vi "总氮通讯.vi"() -> ()   [LabVIEW 2016, in "斯坦道总氮.lvlib"]
uses:
  <vilib>/NI/Modbus Library/API/Wrapper/Create TCP Slave.vi
  <vilib>/Utility/config.llb/Write Key (Boolean).vi
  <vilib>/Utility/config.llb/Write Key (String).vi
  <vilib>/Plasmionique/MB Master/MB_Master/MB_Master.lvclass
  <vilib>/NI/Modbus Library/API/Slave/Modbus Slave.lvclass
  <vilib>/Utility/config.llb/NI_LVConfig.lvlib
  <vilib>/Plasmionique/MB Master/MB Master.lvlib
  <vilib>/NI/Modbus Library/API/Wrapper/API Main.lvlib
panel:
  out "总氮测量数据区":u16[](array[numeric])
  out "总氮状态告警区":u16[](array[numeric])
  out "总磷状态告警区":u16[](array[numeric])
  out "总磷测量数据区":u16[](array[numeric])
  out "序列号":string
  out "状态告警区":T1 {"告警代码" items=["无告警", "缺试剂告警", "缺水样告警", "缺蒸馏水告警", "缺标液告警", "仪表漏液告警", "标定异常告警", "超量程告警", "加热异常", "低试剂预警", "超上限告警", "超下限告警", "仪表内部其他异常", "滴定异常告警", "电极异常告警", "量程切换告警", "参数设置告警", "PH电极电位异常", "电导率电极异常", "浊度光度异常", "溶解氧电极异常", "溶解氧光强异常", "温度异常告警", "PH异常告警", "溶解氧异常告警", "电导率异常告警", "浊度异常告警", "叶绿素异常告警", "藻密度异常告警", "蓝绿藻异常告警", "ORP异常告警", "氨氮异常告警", "清洁刷异常告警", "SD卡异常告警", "蓝牙异常告警", "Wifi异常告警", "流程异常告警"]; "故障代码" items=["无故障", "电机故障", "温度故障", "通讯故障", "滴定故障"]}
  out "测量数据区":T2 {"单位" items=["ug/L", "mg/L", "ppm", "mg/m3", "cm", "ppb", "ug/m3", "%", "nmol/mol", "umol/mol", "MPN/L", "MPN/100ml", "ng/m3", "NTU", "无量纲", "ms/cm", "us/cm", "℃", "mV", "万个/L"]}
  out "status":bool
  out "关键参数区":T3
  in  "读关键参数区":bool
  in  "读状态告警区":bool
  in  "读测量数据区":bool
  in  "站号":u16(ring) items=["总磷"=1, "氨氮"=3]
  in  "停止":bool
  in  "启动":bool
  in  "控制命令":u16(ring) items=["启动测量"=1, "标样核查"=2, "零点核查"=3, "跨度核查"=4, "空白测试"=5, "平行样测试"=6, "加标回收"=7, "空白校准"=8, "标样校准"=9, "初始化（清洗）"=10, "停止测试"=11, "仪器重启"=12, "校时"=13, "模式设置"=14, "测量间隔设置"=15]
  in  "控制命令参数":u16[](array[numeric]) format="%04xH"
  in  "VISA Resource":refnum<visa-resource-name>
  in  "启用模块":bool
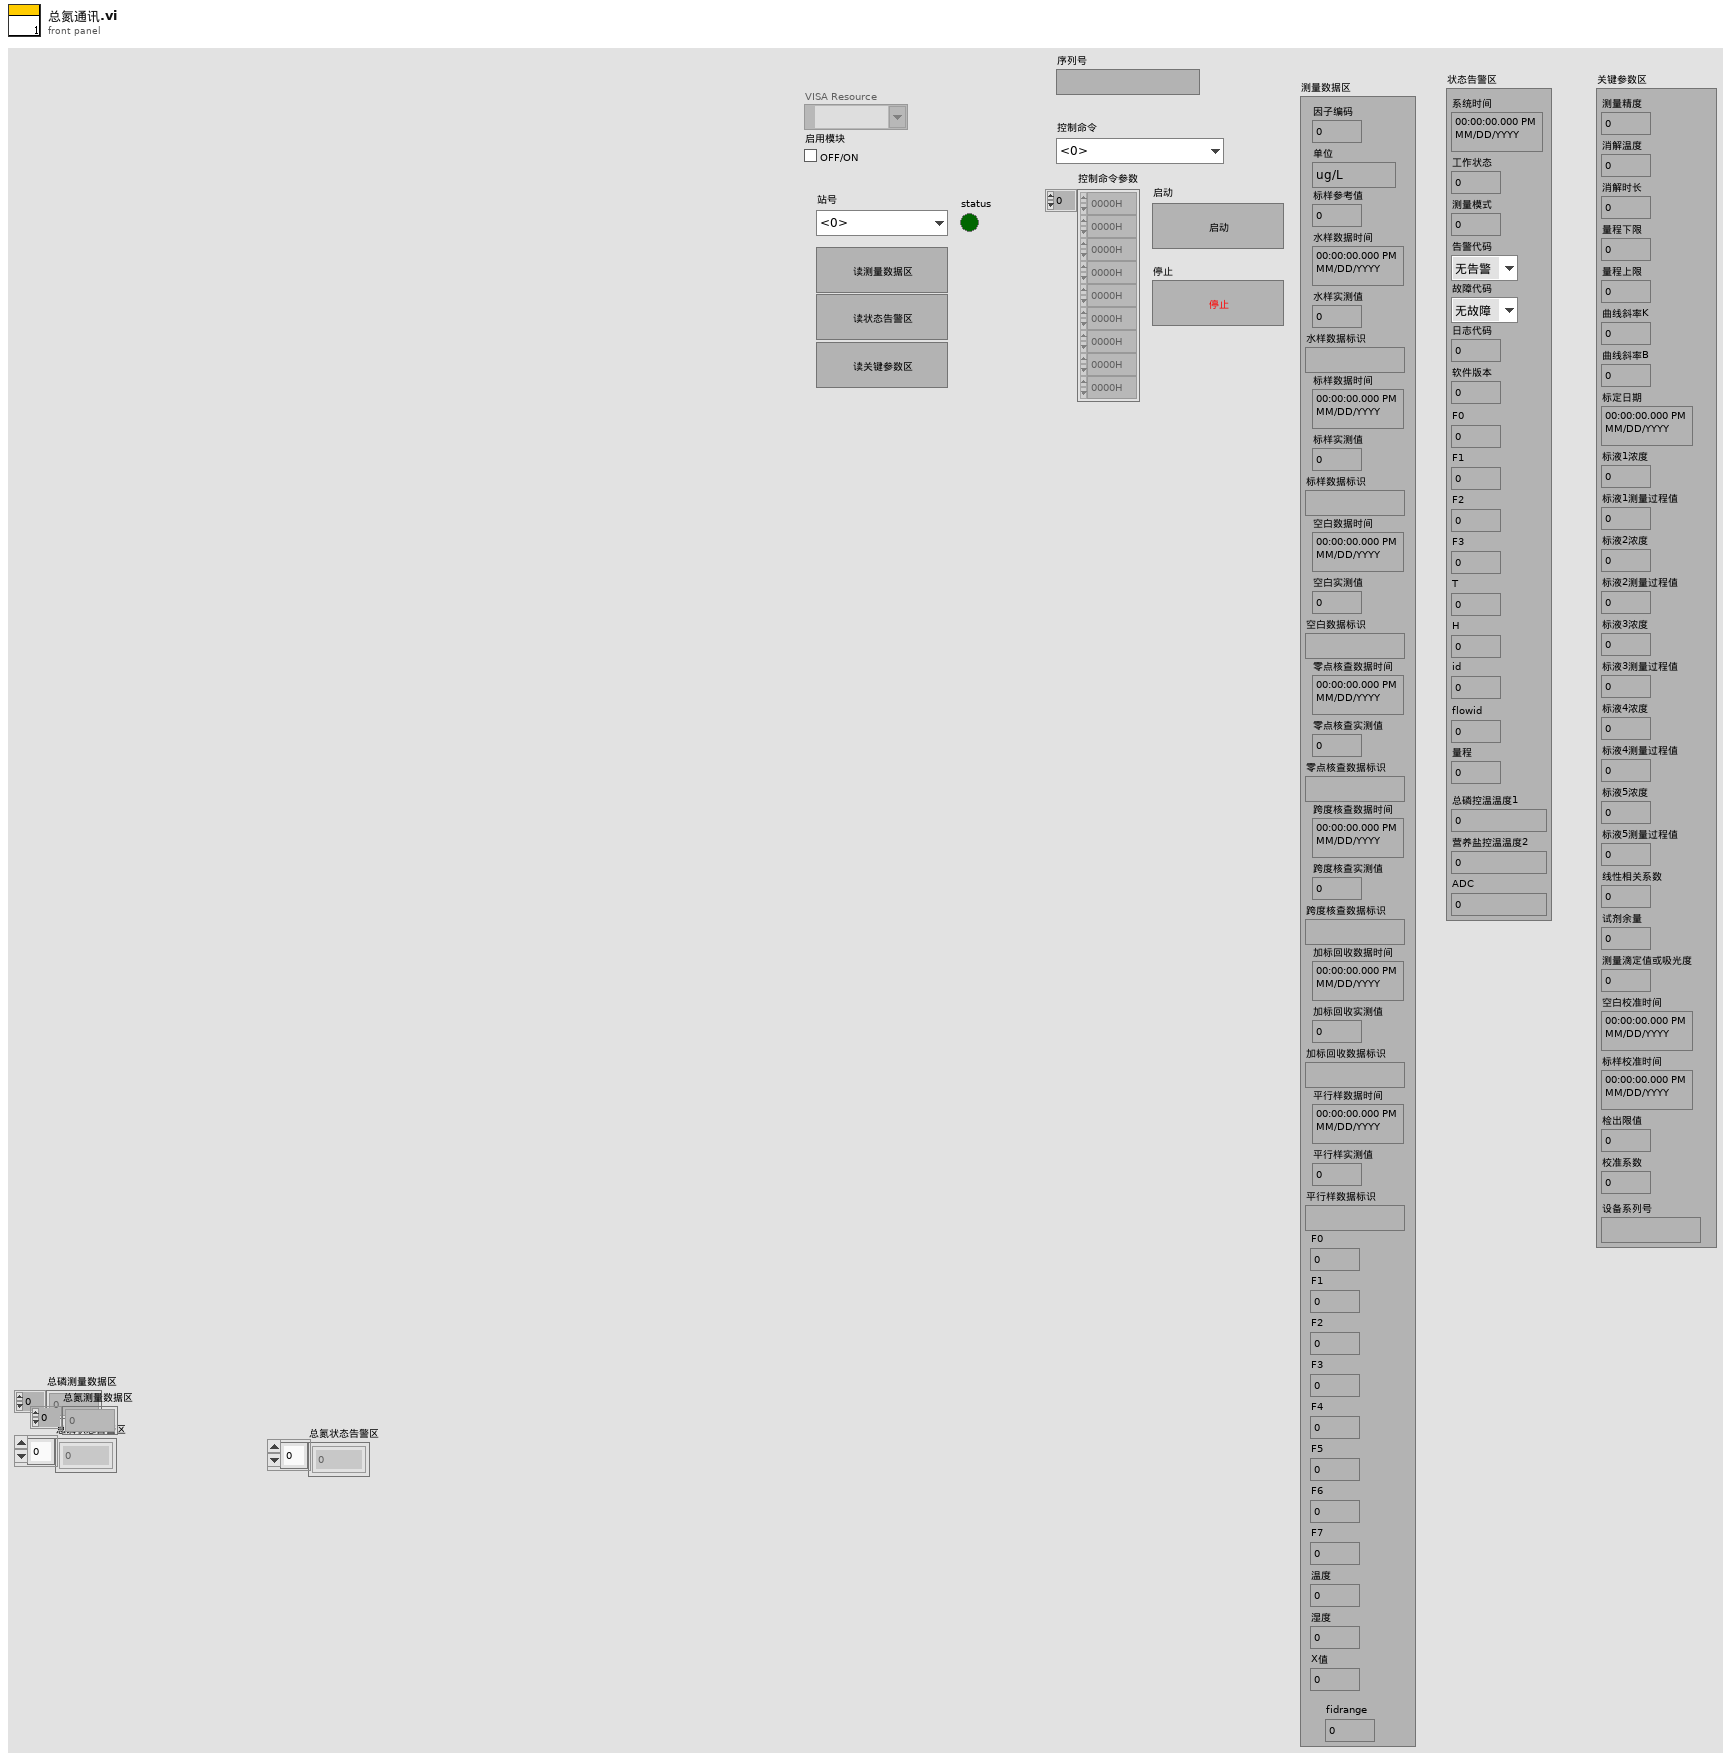
[diagram p1: front panel]
types:
  T1 = cluster{"系统时间":timestamp, "工作状态":u16, "测量模式":u16, "告警代码":u16, "故障代码":u16, "日志代码":u16, "软件版本":u16, "F0":sgl, "F1":sgl, "F2":sgl, "F3":sgl, "T":sgl, "H":sgl, "id":u16, "flowid":u16, "量程":u16, "总磷控温温度1":sgl, "营养盐控温温度2":sgl, "ADC":sgl}
  T2 = cluster{"因子编码":u32, "单位":u16, "标样参考值":sgl, "水样数据时间":timestamp, "水样实测值":sgl, "水样数据标识":string, "标样数据时间":timestamp, "标样实测值":sgl, "标样数据标识":string, "空白数据时间":timestamp, "空白实测值":sgl, "空白数据标识":string, "零点核查数据时间":timestamp, "零点核查实测值":sgl, "零点核查数据标识":string, "跨度核查数据时间":timestamp, "跨度核查实测值":sgl, "跨度核查数据标识":string, "加标回收数据时间":timestamp, "加标回收实测值":sgl, "加标回收数据标识":string, "平行样数据时间":timestamp, "平行样实测值":sgl, "平行样数据标识":string, "F0":sgl, "F1":sgl, "F2":sgl, "F3":sgl, "F4":sgl, "F5":sgl, "F6":sgl, "F7":sgl, "温度":sgl, "湿度":sgl, "X值":sgl, "fidrange":u16}
  T3 = cluster{"测量精度":u16, "消解温度":u16, "消解时长":u16, "量程下限":sgl, "量程上限":sgl, "曲线斜率K":sgl, "曲线斜率B":sgl, "标定日期":timestamp, "标液1浓度":sgl, "标液1测量过程值":sgl, "标液2浓度":sgl, "标液2测量过程值":sgl, "标液3浓度":sgl, "标液3测量过程值":sgl, "标液4浓度":sgl, "标液4测量过程值":sgl, "标液5浓度":sgl, "标液5测量过程值":sgl, "线性相关系数":sgl, "试剂余量":u32, "测量滴定值或吸光度":sgl, "空白校准时间":timestamp, "标样校准时间":timestamp, "检出限值":sgl, "校准系数":sgl, "设备系列号":string}
  T4 = cluster{"水样测试量程模式":enum16{"H", "L", "AUTO"}, "空白核查量程模式":enum16{"H", "L", "AUTO"}, "跨度核查量程模式":enum16{"H", "L", "AUTO"}, "加标回收量程模式":enum16{"H", "L", "AUTO"}}
  T5 = typedef "NI_LVConfig.lvlib/Config Data RefNum.ctl" = refnum<k1>
  T6 = enum8{"Enabled", "Disabled", "Disabled and Grayed Out"}
  T7 = cluster{"系统时间":timestamp, "工作状态":enum16{"空闲", "水样测试", "标样核查", "零点核查", "跨度核查", "空白测试", "平行样测试", "加标回收", "空白校准", "标样校准", "初始化（清洗）"}, "测量模式":enum16{"待机", "连续模式", "周期模式", "定点模式", "受控模式", "手动模式"}, "告警代码":u16, "故障代码":u16, "日志代码":u16, "软件版本":u16, "F0":sgl, "F1":sgl, "F2":sgl, "F3":sgl, "T":sgl, "H":sgl, "id":u16, "flowid":u16, "量程":u16, "总磷控温温度1":sgl, "营养盐控温温度2":sgl, "ADC":sgl}
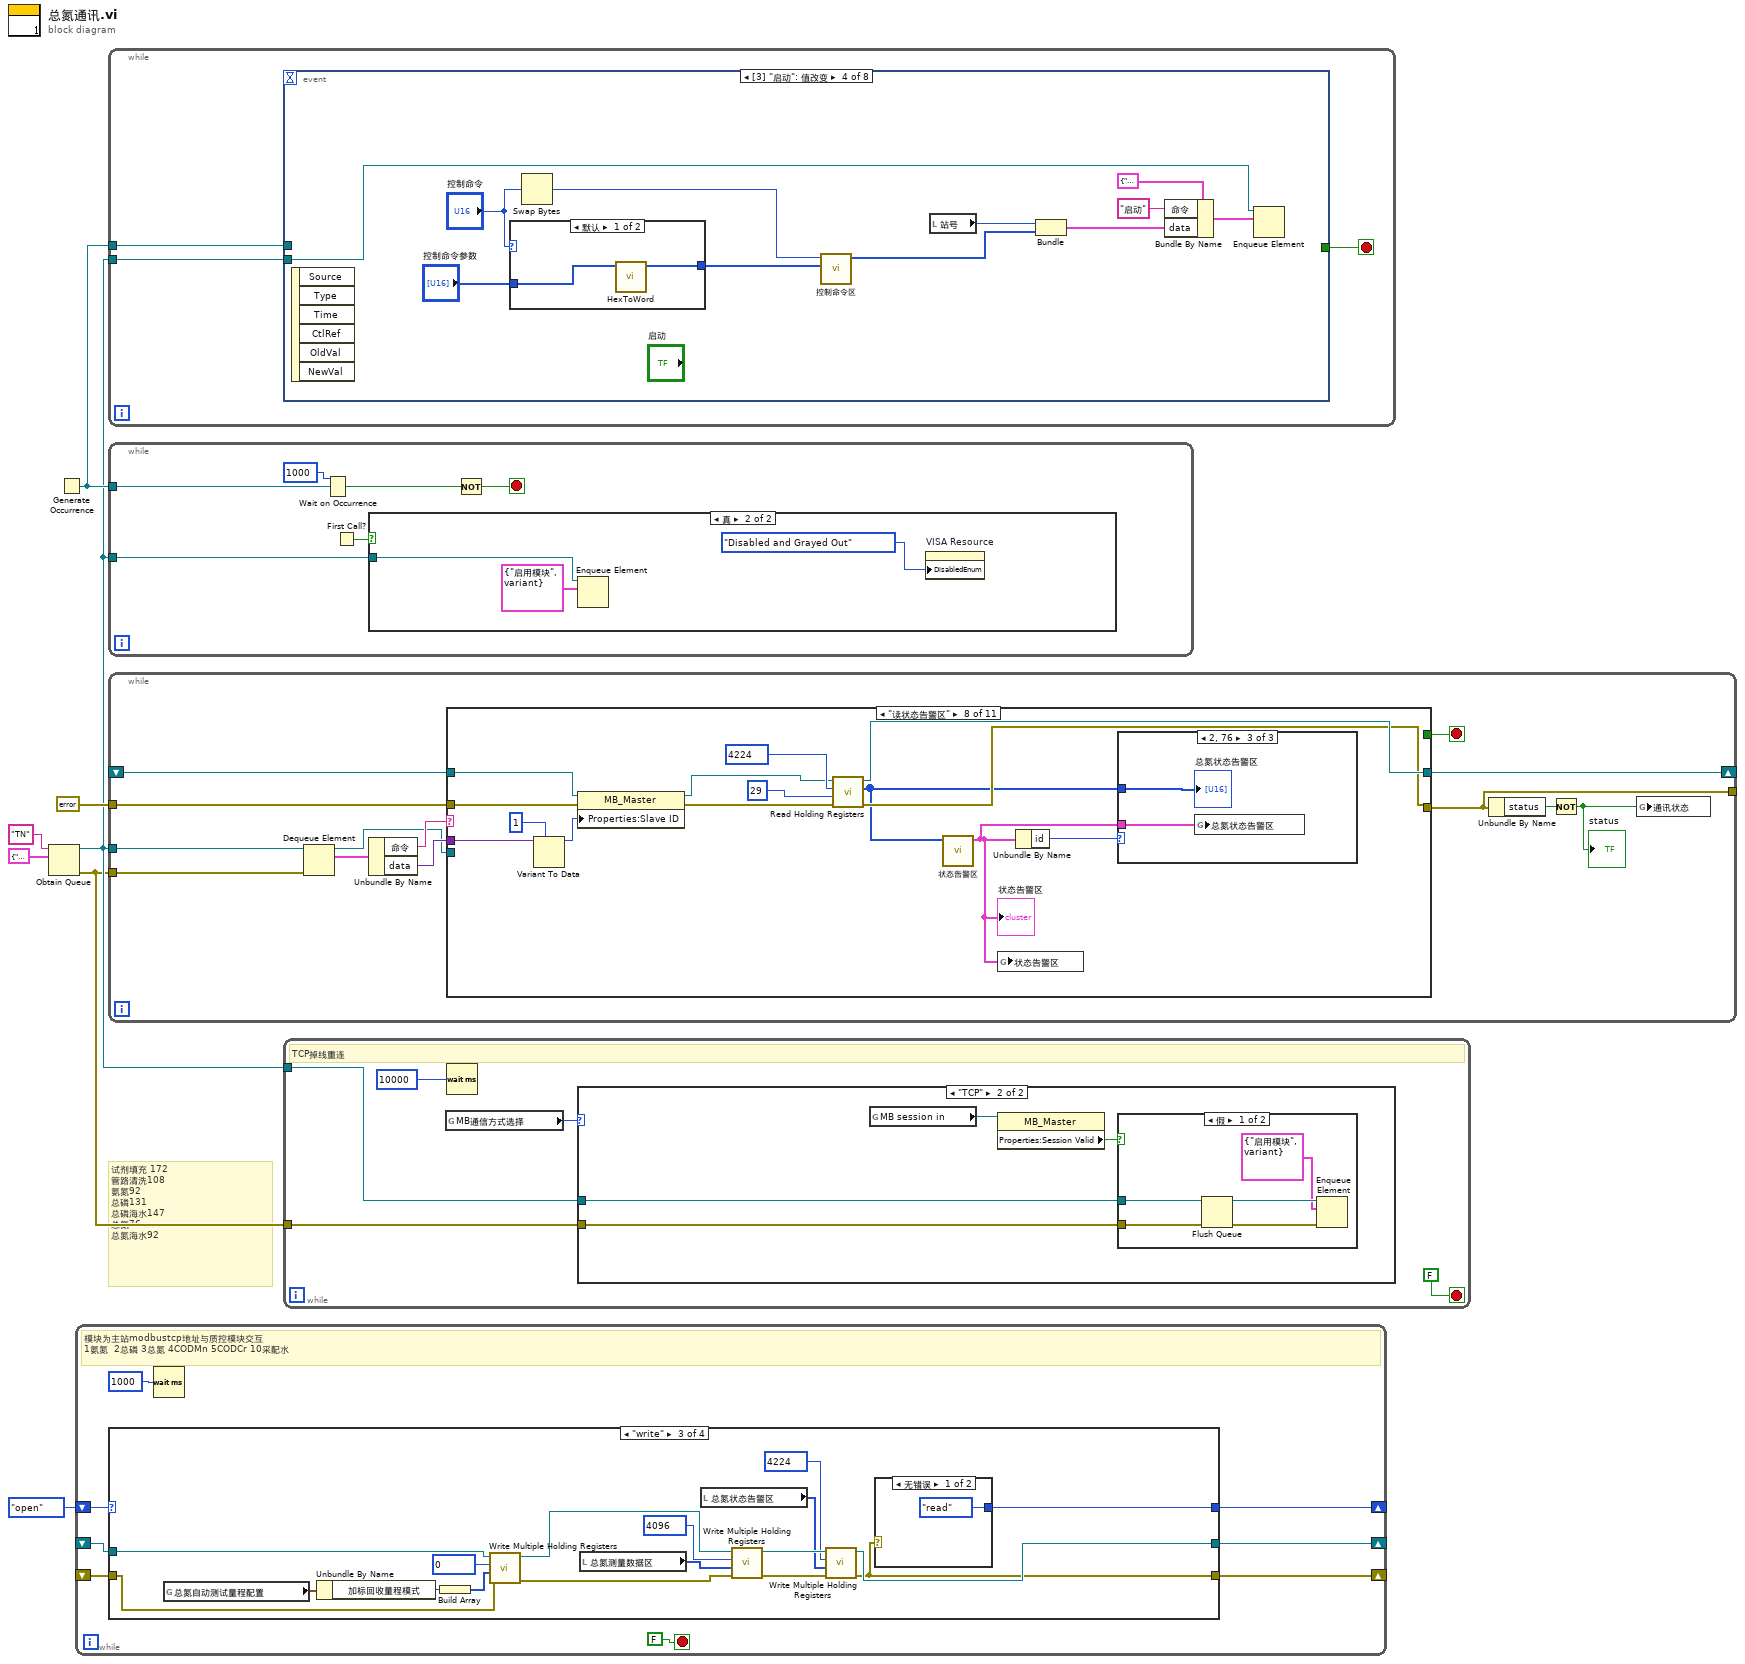
[diagram p0: block diagram]
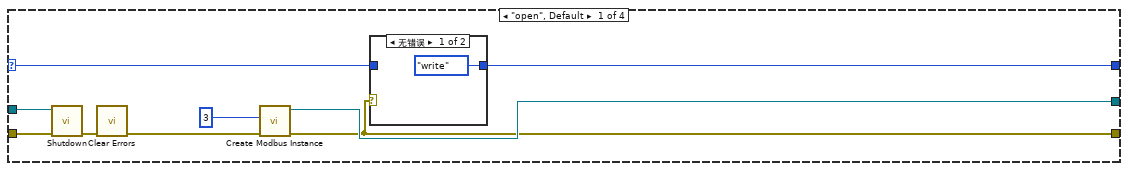
[diagram p4: hidden frame]
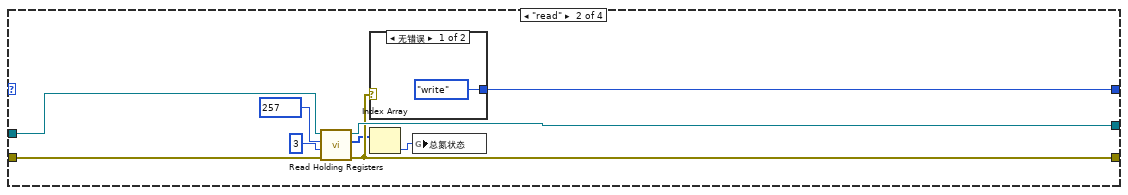
[diagram p6: hidden frame]
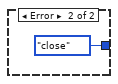
[diagram p7: hidden frame]
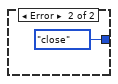
[diagram p8: hidden frame]
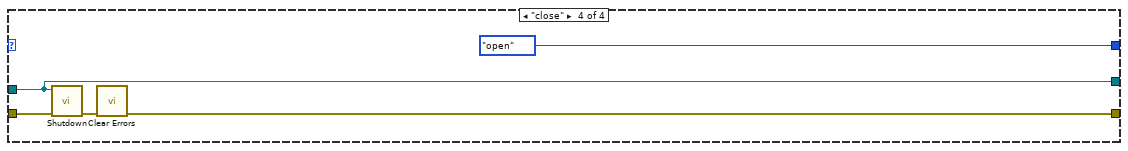
[diagram p9: hidden frame]
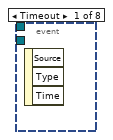
[diagram p11: hidden frame]
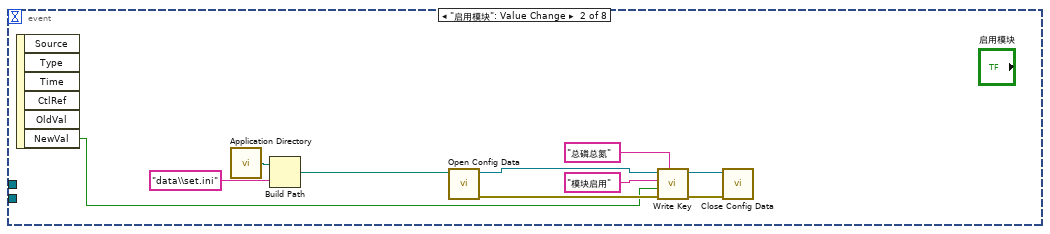
[diagram p12: hidden frame]
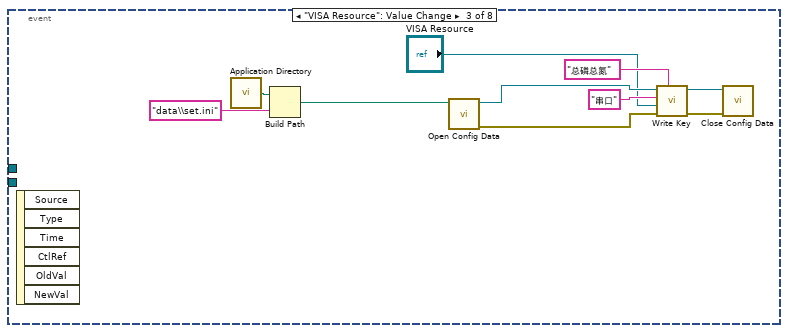
[diagram p13: hidden frame]
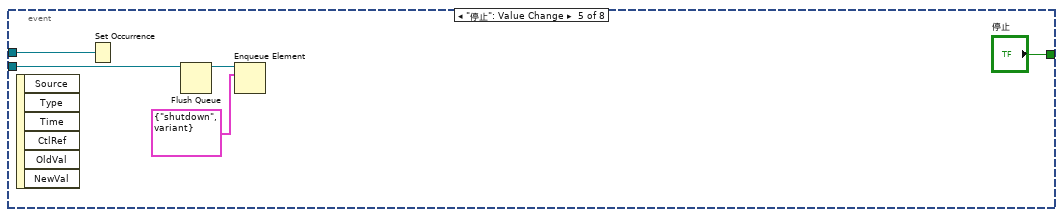
[diagram p15: hidden frame]
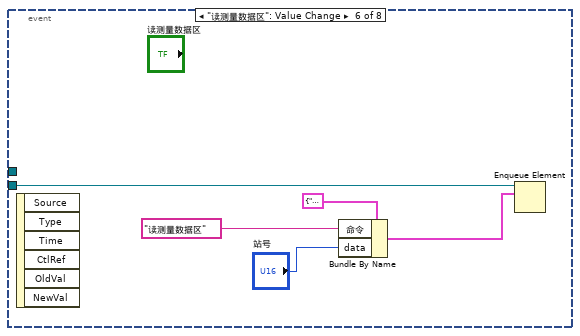
[diagram p16: hidden frame]
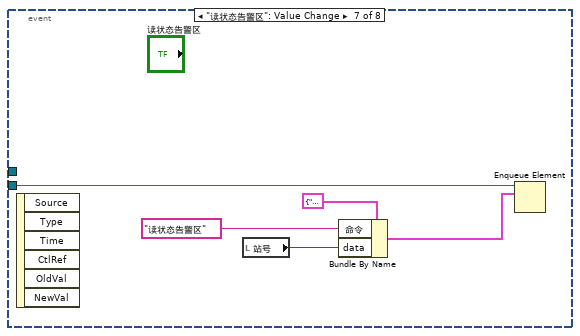
[diagram p17: hidden frame]
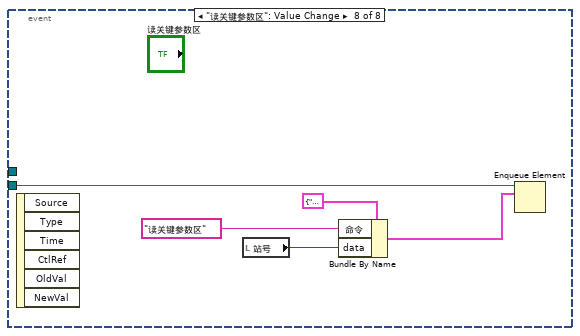
[diagram p18: hidden frame]
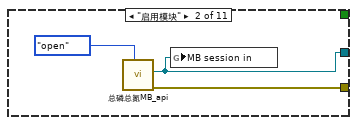
[diagram p20: hidden frame]
diagram:
  # "试剂填充 172 \n管路清洗108\n氨氮92\n总磷131\n总磷海水147\n总氮76\n总氮海水92"
  n1 = Obtain Queue(name (unnamed)="TN" ("名称（未命名）"), element data type=cluster{"命令":string, "data":variant} {"命令"="", "data"=variant}) -> (queue out=w2:refnum<queue>, error out=w1:errorcluster)  [unwired: 3 in, 1 out]
  n2 = Generate Occurrence() -> (w4:refnum<k4>)
  n3 = while {
    shift-right: [w13] -> _
    shift-left: _ -> [w15]
    shift-right: [w12] -> _
    shift-left: _ -> [w14]
    shift-right: [w9] -> _
    shift-left: enum16{"open", "read", "write", "close"}."open" -> [w10]
    stop <- FALSE stop-if-true
    # "模块为主站modbustcp地址与质控模块交互\n1氨氮  2总磷 3总氮 4CODMn 5CODCr 10采配水"
    n4 = case shown="\"write\"" w10 {
      selector: w10 -> [w24 _ _ _]
      tunnel: w15 -> [w18 w34 w41 w59]
      tunnel: w14 -> [w17 w33 w40 w58]
      tunnel: [w21 w30 w50 w59] -> w13
      tunnel: [w20 w29 w49 w61] -> w12
      tunnel: [w23 w35 w54 enum16{"open", "read", "write", "close"}."open"] -> w9
      frame "open", Default {
        n5 = call-dynamic "Shutdown.vi"("error in"=w17, "Modbus slave in"=w18) -> ("error out"=w16:errorcluster)  [unwired: 9 in]
        n6 = call <vilib>:"Clear Errors.vi"("error in (no error)"=w16) -> ("error out"=w19:errorcluster)  [unwired: 5 in, 1 out]
        n7 = call-poly <vilib>:"Create Modbus Instance.vi"("error in"=w19, "port (502)"=u16 3) -> ("error out"=w20:errorcluster, "TCP slave instance"=w21:refnum<class "Modbus Slave.lvclass">)  [unwired: 8 in]
        n8 = case shown="无错误" w20 {
          tunnel: w24 -> [_ w26]
          tunnel: [enum16{"open", "read", "write", "close"}."write" w26] -> w23
          frame No Error {
          }
          frame Error {
          }
        }
      }
      frame "read" {
        n9 = call-dynamic <vilib>:"Read Holding Registers.vi"("error in"=w33, "number of inputs"=u16 3, "starting address"=u16 257, "Modbus slave in"=w34) -> ("error out"=w29:errorcluster, "register values"=w28:u16[], "Modbus slave out"=w30:refnum<class "Modbus Slave.lvclass">)  [unwired: 5 in]
        n10 = case shown="无错误" w29 {
          tunnel: [enum16{"open", "read", "write", "close"}."write" enum16{"open", "read", "write", "close"}."close"] -> w35
          frame No Error {
          }
          frame Error {
          }
        }
        n11 = Index Array(array=w28) -> (element=w27:u16)  [unwired: 1 in]
        n12 = global write "VAR总氮全局变量.vi" "总氮状态"(w27) -> ()
      }
      frame "write" {
        n13 = global read "总氮断电保存全局变量.vi" "总氮自动测试量程配置"() -> (w43:T4)
        n14 = Unbundle By Name(w43) -> ("加标回收量程模式"=w44:enum16{"H", "L", "AUTO"})
        n15 = Build Array(w44) -> (w42:enum16{"H", "L", "AUTO"}[])
        n16 = call-dynamic "Write Multiple Holding Registers.vi"("error in"=w40, "registers to write"=w42, "starting address"=u16 0, "Modbus slave in"=w41) -> ("error out"=w38:errorcluster, "Modbus slave out"=w39:refnum<class "Modbus Slave.lvclass">)  [unwired: 6 in]
        n17 = local read "总氮测量数据区"() -> (w48:u16[])
        n18 = local read "总氮状态告警区"() -> (w46:u16[])
        n19 = call-dynamic "Write Multiple Holding Registers.vi"("error in"=w38, "registers to write"=w48, "starting address"=u16 4096, "Modbus slave in"=w39) -> ("error out"=w51:errorcluster, "Modbus slave out"=w52:refnum<class "Modbus Slave.lvclass">)  [unwired: 6 in]
        n20 = call-dynamic "Write Multiple Holding Registers.vi"("error in"=w51, "registers to write"=w46, "starting address"=u16 4224, "Modbus slave in"=w52) -> ("error out"=w49:errorcluster, "Modbus slave out"=w50:refnum<class "Modbus Slave.lvclass">)  [unwired: 6 in]
        n21 = case shown="无错误" w49 {
          tunnel: [enum16{"open", "read", "write", "close"}."read" enum16{"open", "read", "write", "close"}."close"] -> w54
          frame No Error {
          }
          frame Error {
          }
        }
      }
      frame "close" {
        n22 = call-dynamic "Shutdown.vi"("error in"=w58, "Modbus slave in"=w59) -> ("error out"=w57:errorcluster)  [unwired: 9 in]
        n23 = call <vilib>:"Clear Errors.vi"("error in (no error)"=w57) -> ("error out"=w61:errorcluster)  [unwired: 5 in, 1 out]
      }
    }
    n24 = Wait (ms)(milliseconds to wait=u32 1000 ("等待时间（毫秒）")) -> ()  [unwired: 1 out]
  }
  n25 = while {
    tunnel: w2 -> [w64]
    tunnel: w4 -> [w62]
    stop <- w63 stop-if-true
    n26 = event shown="[3] \"启动\": 值改变" {
      selector: _ -> [_ _ _ _ _ _ _ _]
      dyn-events: _ -> [_ _ _ _ _ _ _ _]
      timeout: _ -> [_ _ _ _ _ _ _ _]
      tunnel: w64 -> [_ _ _ w95 w102 w108 w113 w118]
      tunnel: [_ _ _ _ "停止" _ _ _] -> w63
      tunnel: w62 -> [_ _ _ _ w99 _ _ _]
      event Timeout {
        n27 = event-data() -> ()  [unwired: 1 in, 3 out]
      }
      event "启用模块": Value Change {
        n28 = event-data() -> ("NewVal"=w65:bool)  [unwired: 1 in, 5 out]
        n29 = call <vilib>:"Application Directory.vi"() -> ("Application Directory"=w67:path)
        n30 = Build Path(base path=w67, name or relative path="data\\set.ini" ("名称或相对路径")) -> (appended path=w68:path)
        n31 = call <vilib>:"Open Config Data.vi"("configuration file path"=w68) -> ("error out"=w74:errorcluster, "refnum"=w73:T5)  [unwired: 8 in, 1 out]
        n32 = call-poly <vilib>:"Write Key.vi"("section"="总磷总氮", "error in (no error)"=w74, "value"=w65, "key"="模块启用", "refnum"=w73) -> ("error out"=w70:errorcluster, "refnum out"=w66:T5)  [unwired: 4 in, 1 out]
        n33 = call <vilib>:"Close Config Data.vi"("error in (no error)"=w70, "refnum"=w66) -> ()  [unwired: 8 in, 2 out]
      }
      event "VISA Resource": Value Change {
        n34 = event-data() -> ()  [unwired: 1 in, 6 out]
        n35 = call <vilib>:"Application Directory.vi"() -> ("Application Directory"=w77:path)
        n36 = Build Path(base path=w77, name or relative path="data\\set.ini" ("名称或相对路径")) -> (appended path=w78:path)
        n37 = call <vilib>:"Open Config Data.vi"("configuration file path"=w78) -> ("error out"=w84:errorcluster, "refnum"=w83:T5)  [unwired: 8 in, 1 out]
        n38 = call-poly <vilib>:"Write Key.vi"("section"="总磷总氮", "error in (no error)"=w84, "value"="VISA Resource", "key"="串口", "refnum"=w83) -> ("error out"=w80:errorcluster, "refnum out"=w76:T5)  [unwired: 4 in, 1 out]
        n39 = call <vilib>:"Close Config Data.vi"("error in (no error)"=w80, "refnum"=w76) -> ()  [unwired: 8 in, 2 out]
      }
      event "启动": Value Change {
        n40 = event-data() -> ()  [unwired: 1 in, 6 out]
        n41 = case shown="默认" "控制命令" {
          tunnel: "控制命令参数" -> [w97 w98]
          tunnel: [w96 w98] -> w85
          frame Default {
            n42 = call "HexToWord.vi"("数组"=w97) -> ("WORD"=w96:u16[])  [unwired: 10 in]
          }
          frame 13 {
          }
        }
        n43 = Swap Bytes(anything="控制命令") -> (byte swapped=w88:u16)
        n44 = call "控制命令区.vi"("控制命令参数"=w85, "控制命令"=w88) -> ("控制命令"=w91:u16[])  [unwired: 9 in]
        n45 = local read "站号"() -> (w90:u16)
        n46 = Bundle("站号"=w90, "控制命令"=w91) -> (w89:cluster{"站号":u16, "控制命令":u16[]})  [unwired: 1 in]
        n47 = Bundle By Name(cluster=cluster{"命令":string, "data":variant} {"命令"="", "data"=variant} ("元素"), "命令"="启动", "data"=w89) -> (w93:cluster{"命令":string, "data":variant})
        n48 = Enqueue Element(queue=w95, element=w93) -> ()  [unwired: 2 in, 3 out]
      }
      event "停止": Value Change {
        n49 = event-data() -> ()  [unwired: 1 in, 6 out]
        n50 = Set Occurrence(w99) -> ()
        n51 = Flush Queue(queue=w102) -> (queue out=w101:refnum<queue>)  [unwired: 1 in, 2 out]
        n52 = Enqueue Element(queue=w101, element=cluster{"命令":string, "data":variant} {"命令"="shutdown", "data"=variant} ("元素")) -> ()  [unwired: 2 in, 3 out]
      }
      event "读测量数据区": Value Change {
        n53 = event-data() -> ()  [unwired: 1 in, 6 out]
        n54 = Bundle By Name(cluster=cluster{"命令":string, "data":variant} {"命令"="", "data"=variant} ("元素"), "命令"="读测量数据区", "data"="站号") -> (w106:cluster{"命令":string, "data":variant})
        n55 = Enqueue Element(queue=w108, element=w106) -> ()  [unwired: 2 in, 3 out]
      }
      event "读状态告警区": Value Change {
        n56 = event-data() -> ()  [unwired: 1 in, 6 out]
        n57 = local read "站号"() -> (w109:u16)
        n58 = Bundle By Name(cluster=cluster{"命令":string, "data":variant} {"命令"="", "data"=variant} ("元素"), "命令"="读状态告警区", "data"=w109) -> (w111:cluster{"命令":string, "data":variant})
        n59 = Enqueue Element(queue=w113, element=w111) -> ()  [unwired: 2 in, 3 out]
      }
      event "读关键参数区": Value Change {
        n60 = event-data() -> ()  [unwired: 1 in, 6 out]
        n61 = local read "站号"() -> (w114:u16)
        n62 = Bundle By Name(cluster=cluster{"命令":string, "data":variant} {"命令"="", "data"=variant} ("元素"), "命令"="读关键参数区", "data"=w114) -> (w116:cluster{"命令":string, "data":variant})
        n63 = Enqueue Element(queue=w118, element=w116) -> ()  [unwired: 2 in, 3 out]
      }
    }
  }
  n64 = while {
    tunnel: w4 -> [w124]
    tunnel: w2 -> [w120]
    stop <- w121 stop-if-true
    n65 = Wait on Occurrence(2:w124, 3:1000 ("毫秒超时(-1)")) -> (0:w122:bool)  [unwired: 1 in]
    n66 = First Call?() -> (First Call?: T/F=w119:bool)
    n67 = case shown="真" w119 {
      tunnel: w120 -> [_ w126]
      frame False {
      }
      frame True {
        n68 = Enqueue Element(queue=w126, element=cluster{"命令":string, "data":variant} {"命令"="启用模块", "data"=variant} ("元素")) -> ()  [unwired: 2 in, 3 out]
        n69 = property on="VISA Resource" class="VISAName"("DisabledEnum"=T6."Disabled and Grayed Out" ("禁用")) -> ()  [unwired: 2 in, 2 out]
      }
    }
    n70 = Not(x=w122) -> (.not. x?=w121:bool)
  }
  n71 = while {
    tunnel: w2 -> [w140]
    tunnel: w1 -> [w139]
    shift-right: [w137] -> _
    shift-left: _ -> [w136]
    tunnel: errorcluster {"status"=FALSE, "code"=0, "source"=""} ("error out") -> [w135]
    tunnel: [w130] -> _
    stop <- w138 stop-if-true
    n72 = Dequeue Element(queue=w140, error in (no error)=w139) -> (queue out=w131:refnum<queue>, element=w133:cluster{"命令":string, "data":variant})  [unwired: 1 in, 2 out]
    n73 = Unbundle By Name(w133) -> ("命令"=w134:string, "data"=w132:variant)
    n74 = case shown="\"读状态告警区\"" w134 {
      tunnel: w132 -> [_ _ _ w159 w170 w187 w197 w211 w229 w243 _]
      tunnel: w131 -> [_ _ _ _ _ _ _ _ _ _ w256]
      tunnel: [_ _ _ _ _ _ _ _ _ _ TRUE] -> w138
      tunnel: [w141 w144 w146 w162 w173 w189 w201 w220 w236 w250 w252] -> w137
      tunnel: [w142 w143 w147 w161 w172 w188 w202 w210 w237 w251 w253] -> w130
      tunnel: w136 -> [w141 _ w146 w158 w169 w186 w196 w214 w232 w246 w252]
      tunnel: w135 -> [w142 _ w149 w155 w166 w183 w194 w215 w233 w247 w254]
      frame Default {
      }
      frame "启用模块" {
        n75 = call "总磷总氮MB_api.vi"("STEP"=enum16{"open", "read", "write", "close"}."open") -> ("error out"=w143:errorcluster, "MB session out"=w144:refnum<class "MB_Master.lvclass">)  [unwired: 8 in, 1 out]
        n76 = global write "VAR总氮全局变量.vi" "MB session in"(w144) -> ()
      }
      frame "停用模块" {
        n77 = call-dynamic "Close Session.vi"("error in (no error)"=w149, "MB session in"=w146) -> ("error out"=w148:errorcluster)  [unwired: 9 in]
        n78 = call <vilib>:"Clear Errors.vi"("error in (no error)"=w148) -> ("error out"=w147:errorcluster)  [unwired: 5 in, 1 out]
      }
      frame "启动" {
        n79 = Variant To Data(type=cluster{"站号":u16, "控制命令":u16[]} {"站号"=0, "控制命令"=[]} ("输出簇"), Variant=w159) -> (data=w153:cluster{"站号":u16, "控制命令":u16[]})  [unwired: 1 in, 1 out]
        n80 = Unbundle By Name(w153) -> ("站号"=w152:u16, "控制命令"=w150:u16[])
        n81 = property class="MB_Master"(reference=w158, error in=w155, "Properties:Slave ID"=w152) -> (reference out=w157:refnum<class "MB_Master.lvclass">, error out=w156:errorcluster)
        n82 = Index Array(array=w150) -> (element=w151:u16)  [unwired: 1 in]
        n83 = global write "VAR总氮全局变量.vi" "控制命令"(w151) -> ()
        n84 = call <vilib>:"Write Multiple Registers.vi"("error in (no error)"=w156, "values"=w150, "starting address"=u16 4608, "MB session in"=w157) -> ("error out"=w161:errorcluster, "MB session out"=w162:refnum<class "MB_Master.lvclass">)  [unwired: 6 in]
      }
      frame "盲样测试" {
        n85 = Variant To Data(type=0, Variant=w170) -> (data=w163:i32)  [unwired: 1 in, 1 out]
        n86 = property class="MB_Master"(reference=w169, error in=w166, "Properties:Slave ID"=w163) -> (reference out=w168:refnum<class "MB_Master.lvclass">, error out=w167:errorcluster)
        n87 = case shown="默认" w163 {
          tunnel: [u16[] [] ("values") u16[] [33539, 0] ("values") u16[] [23555, 0] ("values")] -> w165
          frame Default {
          }
          frame 1 {
            # "总磷盲样测试命令"
          }
          frame 3 {
            # "氨氮盲样测试"
          }
        }
        n88 = call <vilib>:"Write Multiple Registers.vi"("error in (no error)"=w167, "values"=w165, "starting address"=u16 24592, "MB session in"=w168) -> ("error out"=w172:errorcluster, "MB session out"=w173:refnum<class "MB_Master.lvclass">)  [unwired: 6 in]
      }
      frame "debug" {
        n89 = Variant To Data(type=cluster{"站号":u16, "控制命令":u16[]} {"站号"=0, "控制命令"=[]} ("输出簇"), Variant=w187) -> (data=w181:cluster{"站号":u16, "控制命令":u16[]})  [unwired: 1 in, 1 out]
        n90 = Unbundle By Name(w181) -> ("站号"=w180:u16, "控制命令"=w178:u16[])
        n91 = property class="MB_Master"(reference=w186, error in=w183, "Properties:Slave ID"=w180) -> (reference out=w185:refnum<class "MB_Master.lvclass">, error out=w184:errorcluster)
        n92 = Index Array(array=w178) -> (element=w179:u16)  [unwired: 1 in]
        n93 = global write "VAR总氮全局变量.vi" "控制命令"(w179) -> ()
        n94 = call <vilib>:"Write Multiple Registers.vi"("error in (no error)"=w184, "values"=w178, "starting address"=u16 24594, "MB session in"=w185) -> ("error out"=w188:errorcluster, "MB session out"=w189:refnum<class "MB_Master.lvclass">)  [unwired: 6 in]
      }
      frame "读测量数据区" {
        n95 = Variant To Data(type=u8 1 ("Slave ID"), Variant=w197) -> (data=w192:u8)  [unwired: 1 in, 1 out]
        n96 = property class="MB_Master"(reference=w196, error in=w194, "Properties:Slave ID"=w192) -> (reference out=w195:refnum<class "MB_Master.lvclass">, error out=w193:errorcluster)
        n97 = call <vilib>:"Read Holding Registers.vi"("error in (no error)"=w193, "quantity"=u16 105, "starting address"=u16 4096, "MB session in"=w195) -> ("error out"=w202:errorcluster, "Registers"=w191:u16[], "MB session out"=w201:refnum<class "MB_Master.lvclass">)  [unwired: 5 in]
        n98 = call "测量数据区.vi"("数组"=w191) -> ("测量数据区"=w190:T2)  [unwired: 10 in]
        "测量数据区" <- w190
        n99 = global write "VAR总氮全局变量.vi" "测量数据区"(w190) -> ()
        n100 = case shown="2" w192 {
          tunnel: w190 -> [_ w203 w205]
          tunnel: w191 -> [_ w204 w206]
          frame 0, Default {
          }
          frame 1 {
            n101 = global write "VAR总氮全局变量.vi" "总磷测量数据区"(w203) -> ()
            "总磷测量数据区" <- w204
          }
          frame 2 {
            n102 = global write "VAR总氮全局变量.vi" "总氮测量数据区"(w205) -> ()
            "总氮测量数据区" <- w206
          }
        }
      }
      frame "读状态告警区" {
        n103 = Variant To Data(type=u8 1 ("Slave ID"), Variant=w211) -> (data=w216:u8)  [unwired: 1 in, 1 out]
        n104 = property class="MB_Master"(reference=w214, error in=w215, "Properties:Slave ID"=w216) -> (reference out=w213:refnum<class "MB_Master.lvclass">, error out=w212:errorcluster)
        n105 = call <vilib>:"Read Holding Registers.vi"("error in (no error)"=w212, "quantity"=u16 29, "starting address"=u16 4224, "MB session in"=w213) -> ("error out"=w210:errorcluster, "Registers"=w207:u16[], "MB session out"=w220:refnum<class "MB_Master.lvclass">)  [unwired: 5 in]
        n106 = call "状态告警区.vi"("数组"=w207) -> ("状态告警区"=w208:T7)  [unwired: 10 in]
        "状态告警区" <- w208
        n107 = global write "VAR总氮全局变量.vi" "状态告警区"(w208) -> ()
        n108 = Unbundle By Name(w208) -> ("id"=w209:u16)
        n109 = case shown="2, 76" w209 {
          tunnel: w208 -> [_ w221 w223]
          tunnel: w207 -> [_ w222 w224]
          frame 0, Default {
          }
          frame 1, 131 {
            n110 = global write "VAR总氮全局变量.vi" "总磷状态告警区"(w221) -> ()
            "总磷状态告警区" <- w222
          }
          frame 2, 76 {
            n111 = global write "VAR总氮全局变量.vi" "总氮状态告警区"(w223) -> ()
            "总氮状态告警区" <- w224
          }
        }
      }
      frame "读关键参数区" {
        n112 = Variant To Data(type=u8 1 ("Slave ID"), Variant=w229) -> (data=w227:u8)  [unwired: 1 in, 1 out]
        n113 = property class="MB_Master"(reference=w232, error in=w233, "Properties:Slave ID"=w227) -> (reference out=w231:refnum<class "MB_Master.lvclass">, error out=w230:errorcluster)
        n114 = call <vilib>:"Read Holding Registers.vi"("error in (no error)"=w230, "quantity"=u16 19, "starting address"=u16 4256, "MB session in"=w231) -> ("error out"=w237:errorcluster, "Registers"=w226:u16[], "MB session out"=w236:refnum<class "MB_Master.lvclass">)  [unwired: 5 in]
        n115 = call "关键参数区.vi"("数组"=w226) -> ("关键参数区"=w225:T3)  [unwired: 10 in]
        "关键参数区" <- w225
        n116 = global write "VAR总氮全局变量.vi" "关键参数区"(w225) -> ()
      }
      frame "读序列号" {
        n117 = Variant To Data(type=u8 1 ("Slave ID"), Variant=w243) -> (data=w241:u8)  [unwired: 1 in, 1 out]
        n118 = property class="MB_Master"(reference=w246, error in=w247, "Properties:Slave ID"=w241) -> (reference out=w245:refnum<class "MB_Master.lvclass">, error out=w244:errorcluster)
        n119 = call <vilib>:"Read Holding Registers.vi"("error in (no error)"=w244, "quantity"=u16 6, "starting address"=u16 4, "MB session in"=w245) -> ("error out"=w251:errorcluster, "Registers"=w240:u16[], "MB session out"=w250:refnum<class "MB_Master.lvclass">)  [unwired: 5 in]
        n120 = call "HexToString.vi"("数组"=w240) -> ("STRING"=w239:string[])  [unwired: 10 in]
        n121 = Index Array(array=w239) -> (element=w238:string)  [unwired: 1 in]
        "序列号" <- w238
        n122 = global write "VAR总氮全局变量.vi" "序列号"(w238) -> ()
      }
      frame "shutdown" {
        n123 = call-dynamic "Close Session.vi"("error in (no error)"=w254, "MB session in"=w252) -> ("error out"=w253:errorcluster)  [unwired: 9 in]
        n124 = Flush Queue(queue=w256) -> (queue out=w255:refnum<queue>)  [unwired: 1 in, 2 out]
        n125 = Release Queue(queue=w255) -> ()  [unwired: 2 in, 3 out]
      }
    }
    n126 = Unbundle By Name(w130) -> ("status"=w129:bool)
    n127 = Not(x=w129) -> (.not. x?=w128:bool)
    "status" <- w128
    n128 = global write "VAR总氮全局变量.vi" "通讯状态"(w128) -> ()
  }
  n129 = while "While循环" {
    tunnel: w2 -> [w260]
    tunnel: w1 -> [w259]
    stop <- FALSE stop-if-true
    # "TCP掉线重连"
    n130 = global read "总氮断电保存全局变量.vi" "MB通信方式选择"() -> (w258:enum16{"串口", "TCP"})
    n131 = Wait (ms)(milliseconds to wait=u32 10000 ("等待时间（毫秒）")) -> ()  [unwired: 1 out]
    n132 = case shown="\"TCP\"" w258 {
      tunnel: w260 -> [_ w265]
      tunnel: w259 -> [_ w264]
      frame "串口", Default {
      }
      frame "TCP" {
        n133 = global read "VAR总氮全局变量.vi" "MB session in"() -> (w263:refnum<class "MB_Master.lvclass">)
        n134 = property class="MB_Master"(reference=w263) -> ("Properties:Session Valid"=w266:bool)  [unwired: 1 in, 2 out]
        n135 = case shown="假" w266 {
          tunnel: w265 -> [w269 _]
          tunnel: w264 -> [w268 _]
          frame False {
            n136 = Flush Queue(queue=w269, error in (no error)=w268) -> (queue out=w271:refnum<queue>, error out=w270:errorcluster)  [unwired: 1 out]
            n137 = Enqueue Element(queue=w271, element=cluster{"命令":string, "data":variant} {"命令"="启用模块", "data"=variant} ("元素"), error in (no error)=w270) -> ()  [unwired: 1 in, 3 out]
          }
          frame True {
          }
        }
      }
    }
  }
